vi "Prober_InitialiseUI.vi"(8 "error in (no error)":errorcluster, 11 "AlessiRel6100 in":refnum<class "AlessiRel6100.lvclass">) -> (0 "error out":errorcluster, 2 "Probestation Configuration":variant, 3 "AlessiRel6100 out":refnum<class "AlessiRel6100.lvclass">)   [LabVIEW 2019, in "AlessiRel6100.lvclass"]
uses:
  AlessiRel6100.lvclass
  Alessi.vi
panel:
  in  "Touchdown method":enum16{"no feedback", "Arduino edgesense"}(ring)=enum."Arduino edgesense"
  in  "Overdrive [µm]":i32=30
  in  "Speed [µm/step]":i32=20
  in  "Search Band [µm]":i32=100
  in  "Edgesense params":T1={"touchdown height [µm]"=0, "search band [µm]"=100, "speed [µm/step]"=10, "overdrive [µm]"=30}
  out "Device ID":u32=2
  out "Ref No.":u32
  in  "Needles Clear":bool
  in  "Nucleus":bool
  in  "Stop Button":bool
  # "Starting Probe Station Control Interface"
  # "Arduino Edgesense"
  # "Before continuing, please confirm the following:"
  # "1. NUCLEUS is activiated"
  # "2. No device on chuck and needles are clear"
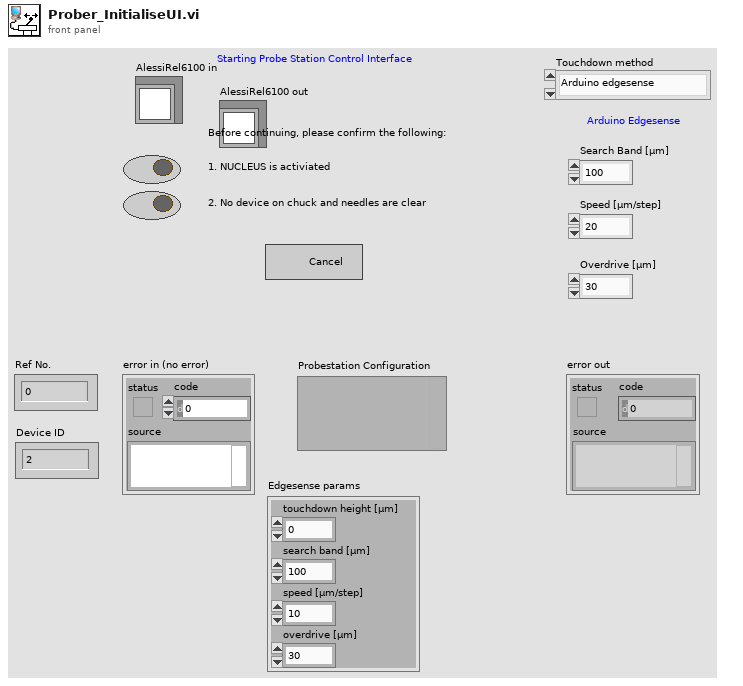
[diagram p1: front panel]
types:
  T1 = cluster{"touchdown height [µm]":i32, "search band [µm]":u32, "speed [µm/step]":u32, "overdrive [µm]":u32}
  T2 = cluster{"Device ID Probe Station":u32, "Ref No.":u32, "Touchdown method":enum16{"no feedback", "Arduino edgesense"}, "Arduino Edgesense params":cluster{"touchdown height [µm]":i32, "search band [µm]":u32, "speed [µm/step]":u32, "overdrive [µm]":u32}}
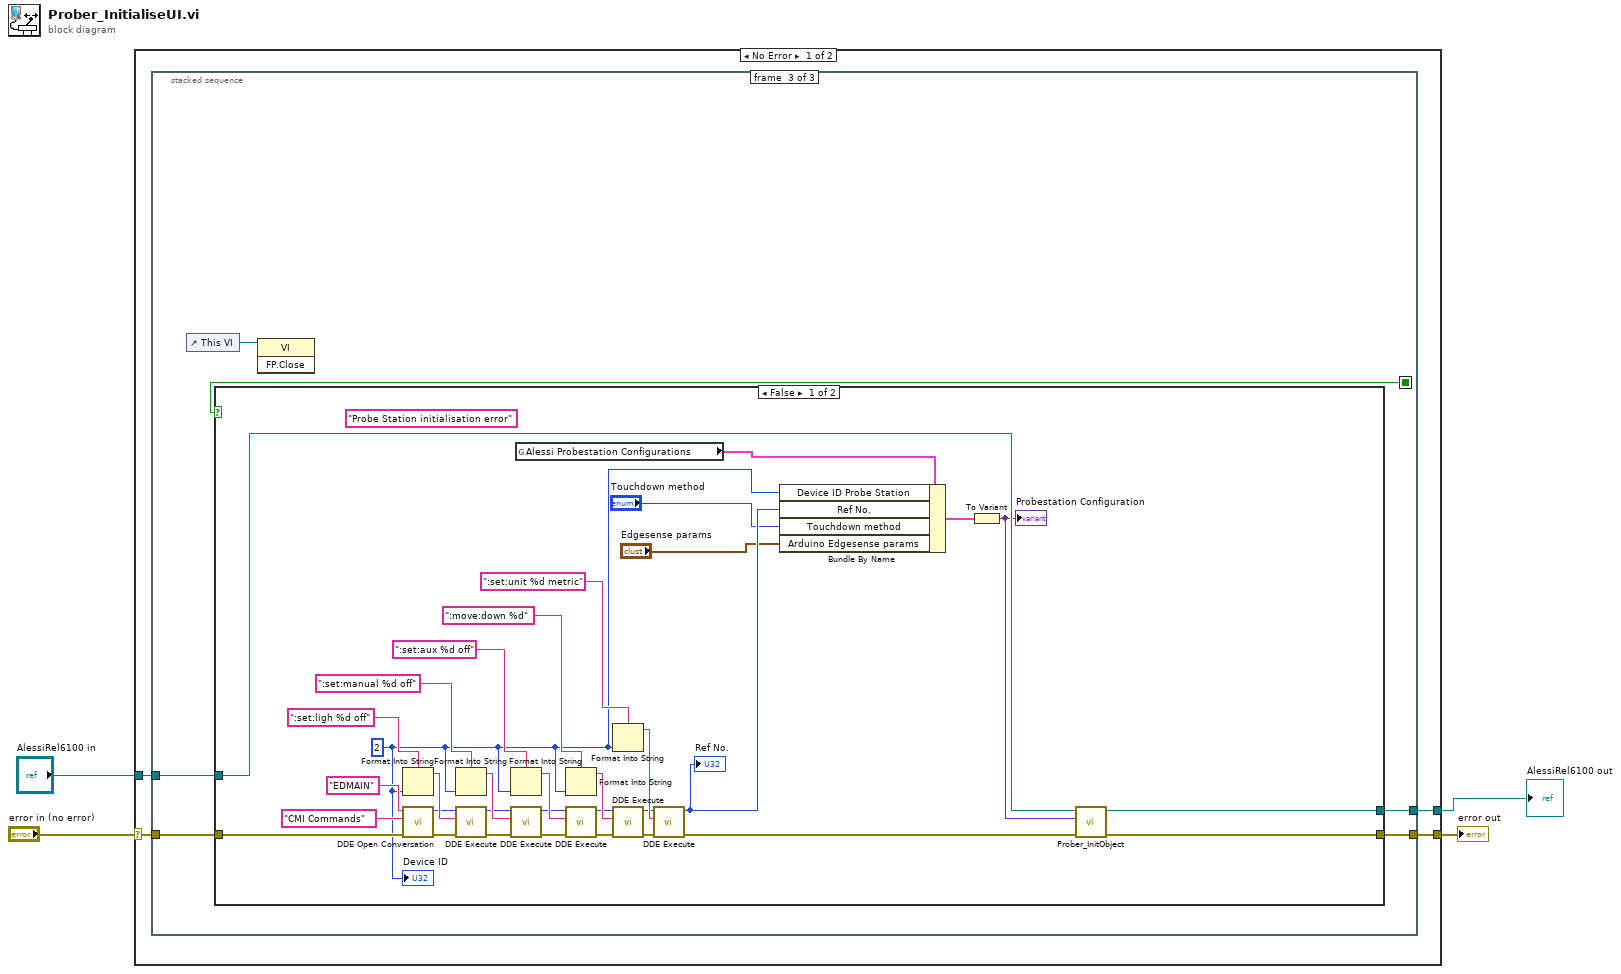
[diagram p0: block diagram]
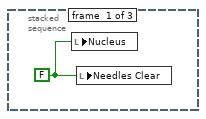
[diagram p2: hidden frame]
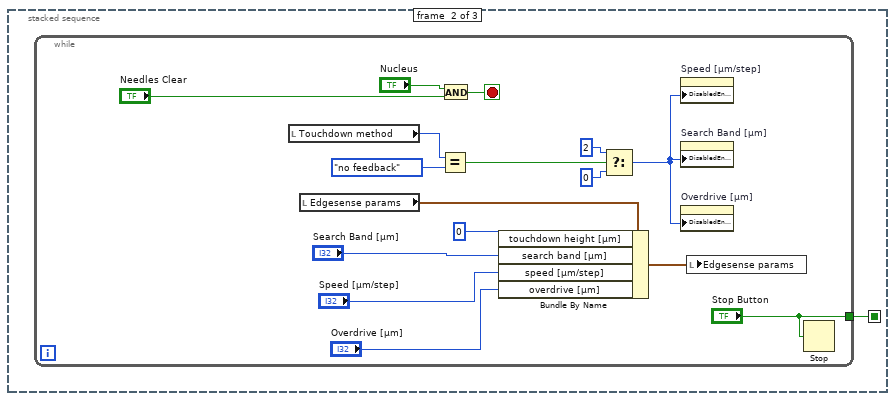
[diagram p3: hidden frame]
diagram:
  n1 = case shown="No Error" "error in (no error)" {
    selector: "error in (no error)" -> [w8 w70]
    tunnel: [w6 w70] -> w2
    tunnel: "AlessiRel6100 in" -> [w7 w69]
    tunnel: [w5 w69] -> w1
    frame No Error {
      n2 = stacked-sequence {
        seq-local: [_ w10 _] -> [_ _ w32]
        tunnel: w8 -> [_ _ w30]
        tunnel: w7 -> [_ _ w31]
        tunnel: [_ _ w29] -> w6
        tunnel: [_ _ w28] -> w5
        frame #0 {
          w9 = FALSE
          n3 = local write "Nucleus"(w9) -> ()
          n4 = local write "Needles Clear"(w9) -> ()
        }
        frame #1 {
          n5 = while {
            tunnel: ["Stop Button"] -> w10
            stop <- w26 stop-if-true
            n6 = local read "Touchdown method"() -> (w15:enum16{"no feedback", "Arduino edgesense"})
            n7 = local read "Edgesense params"() -> (w18:T1)
            n8 = Equal?(x=w15, y=enum16{"no feedback", "Arduino edgesense"}."no feedback" ("Touchdown method")) -> (x = y?=w14:bool)
            n9 = And(x="Nucleus", y="Needles Clear") -> (x .and. y?=w26:bool)
            n10 = Bundle By Name(cluster=w18, "touchdown height [µm]"=0, "search band [µm]"="Search Band [µm]", "speed [µm/step]"="Speed [µm/step]", "overdrive [µm]"="Overdrive [µm]") -> (w17:T1)
            n11 = Select(t=2, s=w14, f=0) -> (s? t:f=w11:i32)
            n12 = property on="Speed [µm/step]" class="DigNum (strict)"("DisabledEnum"=w11) -> ()  [unwired: 2 in, 2 out]
            n13 = property on="Search Band [µm]" class="DigNum (strict)"("DisabledEnum"=w11) -> ()  [unwired: 2 in, 2 out]
            n14 = property on="Overdrive [µm]" class="DigNum (strict)"("DisabledEnum"=w11) -> ()  [unwired: 2 in, 2 out]
            n15 = local write "Edgesense params"(w17) -> ()
            n16 = Stop(stop? (T)="Stop Button") -> ()
          }
        }
        frame #2 {
          n17 = control-ref of="This VI"() -> (w27:refnum<vi>)
          n18 = case shown="False" w32 {
            tunnel: w31 -> [w42 w67]
            tunnel: w30 -> [w41 w68]
            tunnel: [w37 w68] -> w29
            tunnel: [w39 w67] -> w28
            frame False {
              w40 = u32 2
              (unwired) "Probe Station initialisation error" ("Error String IN")
              n19 = Format Into String(format string=":set:ligh %d off", w40) -> (resulting string=w62:string)  [unwired: 2 in, 1 out]
              n20 = call <vilib>:"DDE Open Conversation.vi"("error in (no error)"=w41, "topic"="CMI Commands", "service"="EDMAIN") -> ("error out"=w46:errorcluster, "conversation refnum"=w45:u32)  [unwired: 5 in]
              n21 = Format Into String(format string=":set:manual %d off" ("command"), w40) -> (resulting string=w59:string)  [unwired: 2 in, 1 out]
              n22 = call <vilib>:"DDE Execute.vi"("error in (no error)"=w46, "command"=w62, "conversation refnum in"=w45) -> ("error out"=w50:errorcluster, "conversation refnum out"=w47:u32)  [unwired: 5 in]
              n23 = Format Into String(format string=":set:aux %d off" ("command"), w40) -> (resulting string=w60:string)  [unwired: 2 in, 1 out]
              n24 = call <vilib>:"DDE Execute.vi"("error in (no error)"=w50, "command"=w59, "conversation refnum in"=w47) -> ("error out"=w51:errorcluster, "conversation refnum out"=w48:u32)  [unwired: 5 in]
              n25 = global read "Alessi.vi" "Alessi Probestation Configurations"() -> (w34:T2)
              n26 = Format Into String(format string=":move:down %d" ("command"), w40) -> (resulting string=w61:string)  [unwired: 2 in, 1 out]
              n27 = call <vilib>:"DDE Execute.vi"("error in (no error)"=w51, "command"=w60, "conversation refnum in"=w48) -> ("error out"=w52:errorcluster, "conversation refnum out"=w49:u32)  [unwired: 5 in]
              n28 = Format Into String(format string=":set:unit %d metric" ("command"), w40) -> (resulting string=w66:string)  [unwired: 2 in, 1 out]
              n29 = call <vilib>:"DDE Execute.vi"("error in (no error)"=w52, "command"=w61, "conversation refnum in"=w49) -> ("error out"=w63:errorcluster, "conversation refnum out"=w64:u32)  [unwired: 5 in]
              n30 = call <vilib>:"DDE Execute.vi"("error in (no error)"=w63, "command"=w66, "conversation refnum in"=w64) -> ("error out"=w38:errorcluster, "conversation refnum out"=w44:u32)  [unwired: 5 in]
              "Ref No." <- w44
              n31 = Bundle By Name(cluster=w34, "Device ID Probe Station"=w40, "Ref No."=w44, "Touchdown method"="Touchdown method", "Arduino Edgesense params"="Edgesense params") -> (w43:T2)
              n32 = To Variant(anything=w43) -> (Variant=w33:variant)
              "Probestation Configuration" <- w33
              n33 = call-dynamic "Prober_InitObject.vi"("error in (no error)"=w38, "Prober Configuration"=w33, "AlessiRel6100 in"=w42) -> ("error out"=w37:errorcluster, "AlessiRel6100 out"=w39:refnum<class "AlessiRel6100.lvclass">)  [unwired: 7 in]
              "Device ID" <- w40
            }
            frame True {
            }
          }
          n34 = invoke class="VI" method="FP.Close"(reference=w27) -> ()  [unwired: 2 in, 3 out]
        }
      }
    }
    frame Error {
    }
  }
  "error out" <- w2
  "AlessiRel6100 out" <- w1
